vi "WriteTraceItems.vi"(8 "Error In":errorcluster, 9 "Trace Items":T1[](array[typedef])) -> (0 "Error Out":errorcluster)   [LabVIEW 2018, in "TracerLibrary.lvlib" / "Tracer.lvclass"]
uses:
  Tracer.lvclass
  TraceItemDefinition.ctl
  protected/Tracer_ClassAttributes.vi
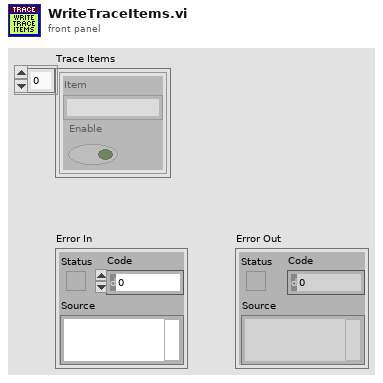
[diagram p1: front panel]
types:
  T1 = typedef "TracerLibrary.lvlib/Tracer.lvclass/TraceItemDefinition.ctl" = cluster{"Item":string, "Enable":bool}
  T2 = typedef "TRACE.lvlib/TRACE.lvclass/TRACE_ObjectAttributes.ctl" = cluster{"TraceContainer":variant}
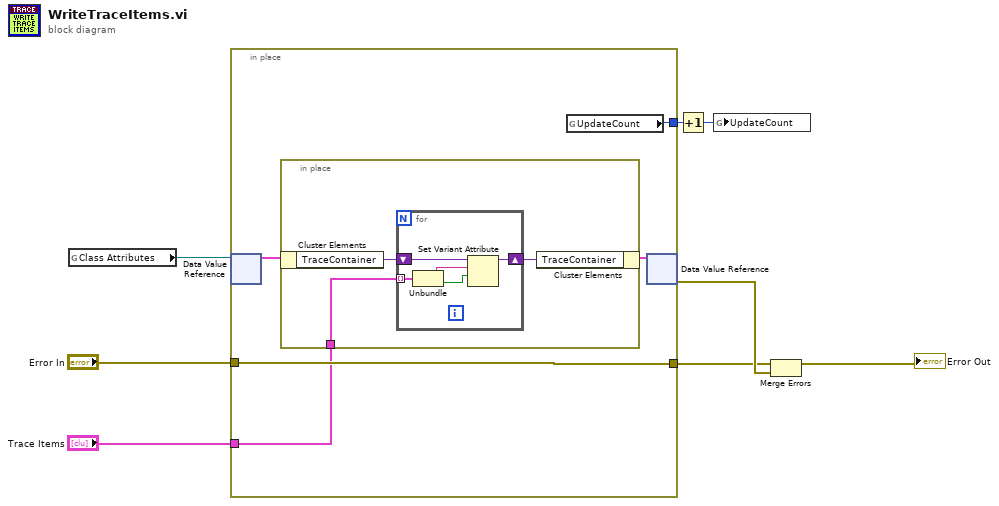
[diagram p0: block diagram]
diagram:
  n1 = global read "Tracer_ClassAttributes.vi" "Class Attributes"() -> (w4:refnum<data-value>)
  n2 = in-place {
    in-place-border: "Error In" -> [w13]
    in-place-border: [w13] -> w5
    in-place-border: "Trace Items" -> [w11]
    in-place-border: [w9] -> w1
    n3 = in-place-dvr #1(w4) -> (w12:T2)  [unwired: 1 out]
    n4 = in-place {
      in-place-border: w11 -> [w14]
      n5 = in-place-cluster #2(w12) -> ("TraceContainer"=w16:variant)
      n6 = for {
        shift-right: [w20] -> w15
        shift-left: w16 -> [w21]
        tunnel: w14 -> [w19] mode=indexing
        n7 = Unbundle(w19) -> ("Item"=w18:string, "Enable"=w17:bool)
        n8 = Set Variant Attribute(Variant=w21, name=w18, value=w17) -> (Variant out=w20:variant)  [unwired: 1 in, 2 out]
      }
      n9 = in-place-cluster #2("TraceContainer"=w15) -> (w10:T2)
    }
    n10 = global read "Tracer_ClassAttributes.vi" "UpdateCount"() -> (w9:i32)
    n11 = in-place-dvr #1(w10) -> (w8:errorcluster)  [unwired: 1 out]
  }
  n12 = Increment(x=w1) -> (x+1=w2:i32)
  n13 = global write "Tracer_ClassAttributes.vi" "UpdateCount"(w2) -> ()
  n14 = Merge Errors(w5, w8) -> (→"Error Out":errorcluster)
